vi "SPI_SetMaxSpeed.vi"(5 "Device":i32, 6 "max speed (Hz)":u32=500000, 7 "Bus":i32=1, 8 "error in":errorcluster) -> (0 "error out":errorcluster)   [LabVIEW 2014, in "GPIO.lvlib"]
doc: "Sets the maximum speed for the specified SPI device, default is 500 kHz."
uses:
  GPIO.lvlib
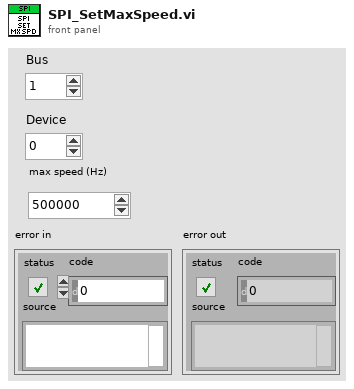
[diagram p1: front panel]
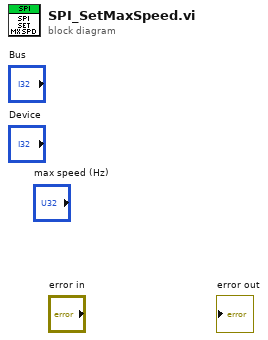
[diagram p0: block diagram]
diagram:
